vi "Settings_init.vi"(2 "error in":errorcluster) -> (0 "error out":errorcluster)   [LabVIEW 2009, in "Utility.lvlib"]
uses:
  Utility.lvlib
  <vilib>/Utility/config.llb/Read Key (String).vi
  <vilib>/Utility/config.llb/NI_LVConfig.lvlib
panel:
  out "appended path":path
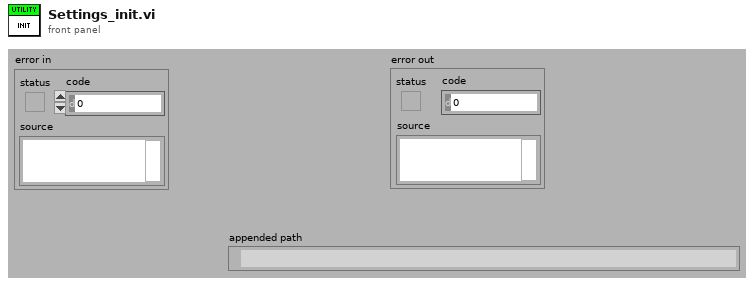
[diagram p1: front panel]
types:
  T1 = typedef "NI_LVConfig.lvlib/Config Data RefNum.ctl" = refnum<k1>
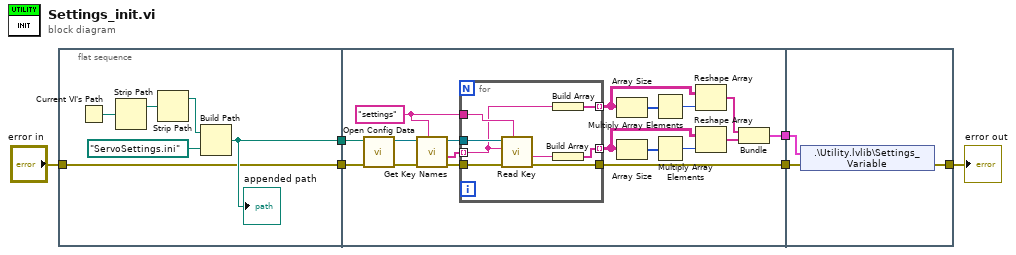
[diagram p0: block diagram]
diagram:
  n1 = flat-sequence {
    tunnel: [w8] -> w6
    tunnel: "error in" -> [w7]
    tunnel: [w7] -> w4
    tunnel: w6 -> [w30]
    tunnel: w4 -> [w29]
    tunnel: [w23] -> w3
    tunnel: [w13] -> w2
    tunnel: w3 -> [w40]
    tunnel: w2 -> [w41]
    tunnel: [w39] -> w1
    frame #0 {
      n2 = Current VI's Path() -> (path=w12:path)
      n3 = Strip Path(path=w12) -> (stripped path=w11:path)  [unwired: 1 out]
      n4 = Strip Path(path=w11) -> (stripped path=w10:path)  [unwired: 1 out]
      n5 = Build Path(base path=w10, name or relative path=path "ServoSettings.ini" ("configuration file path")) -> (appended path=w8:path)
      "appended path" <- w8
    }
    frame #1 {
      w24 = "settings" ("section")
      n6 = call <vilib>:"Open Config Data.vi"("error in (no error)"=w29, "configuration file path"=w30) -> ("error out"=w28:errorcluster, "refnum"=w27:T1)  [unwired: 7 in, 1 out]
      n7 = call <vilib>:"Get Key Names.vi"("section"=w24, "error in (no error)"=w28, "refnum"=w27) -> ("error out"=w26:errorcluster, "key names"=w22:string[], "refnum out"=w25:T1)  [unwired: 5 in, 1 out]
      n8 = for {
        tunnel: w26 -> [w38]
        tunnel: w22 -> [w32] mode=indexing
        tunnel: w25 -> [w37]
        tunnel: w24 -> [w36]
        tunnel: [w34] -> w15 mode=indexing
        tunnel: [w33] -> w23
        tunnel: [w31] -> w19 mode=indexing
        n9 = call-poly <vilib>:"Read Key.vi"("section"=w36, "error in (no error)"=w38, "key"=w32, "refnum"=w37) -> ("error out"=w33:errorcluster, "value"=w35:string)  [unwired: 4 in, 2 out]
        n10 = Build Array(w32) -> (w31:string[])
        n11 = Build Array(w35) -> (w34:string[])
      }
      n12 = Array Size(array=w19) -> (size(s)=w21:i32[])
      n13 = Array Size(array=w15) -> (size(s)=w17:i32[])
      n14 = Multiply Array Elements(1:w21) -> (0:w20:i32)
      n15 = Multiply Array Elements(1:w17) -> (0:w16:i32)
      n16 = Reshape Array(w19, w20) -> (w18:string[])
      n17 = Reshape Array(w15, w16) -> (w14:string[])
      n18 = Bundle(w18, w14) -> (w13:cluster{string[], string[]})  [unwired: 1 in]
    }
    frame #2 {
      n19 = shared-variable ".\\Utility.lvlib\\Settings_Variable"(w41, error in=w40) -> (error out=w39:errorcluster)
    }
  }
  "error out" <- w1
